vi "EXCEL 画曲线.vi"(8 "错误输入（无错误）":errorcluster, 11 "路径":path) -> (0 "error IO":errorcluster, 2 "XY图":cluster{"X":dbl, "Y":dbl}[](graph))   [LabVIEW 2018]
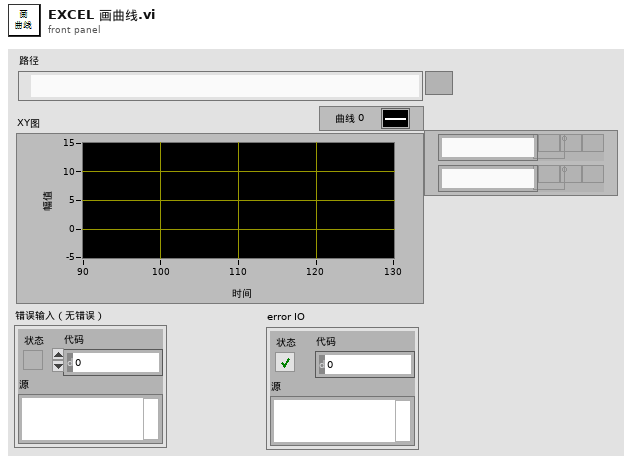
[diagram p1: front panel]
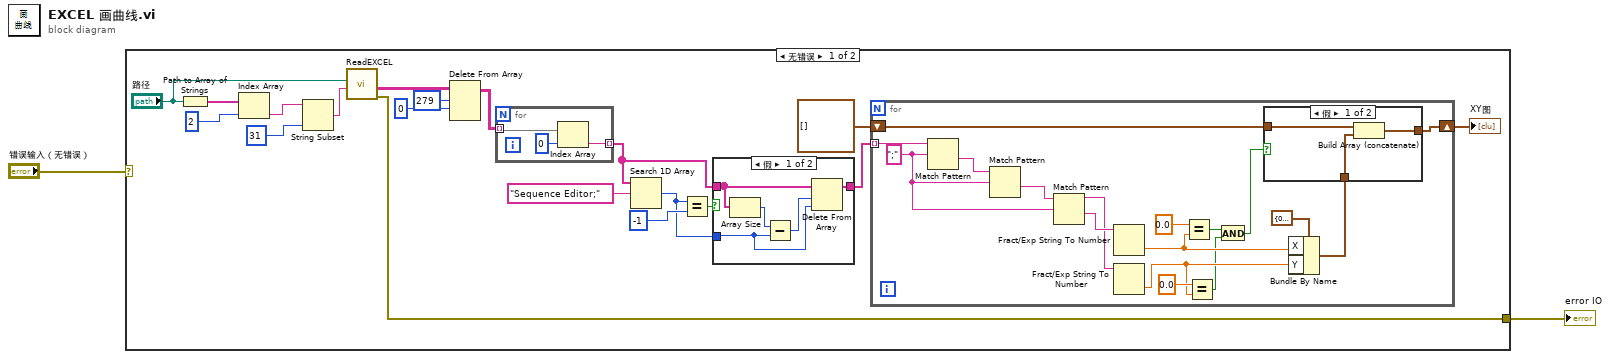
[diagram p0: block diagram]
diagram:
  n1 = case shown="无错误" "错误输入（无错误）" {
    selector: "错误输入（无错误）" -> [_ w52]
    tunnel: [w9 w52] -> w1
    frame No Error {
      n2 = Path to Array of Strings(0:"路径") -> (2:w20:string[])  [unwired: 1 out]
      n3 = Index Array(array=w20, index=2 ("索引")) -> (element=w18:string)
      n4 = String Subset(string=w18, length (rest)=31 ("长度（剩余）")) -> (substring=w16:string)  [unwired: 1 in]
      n5 = call "ReadEXCEL.vi"("EXCEL 标签"=w16, "路径"="路径") -> ("错误输出"=w9:errorcluster, "数据"=w10:string[][])  [unwired: 8 in]
      n6 = Delete From Array(array=w10, length=279 ("长度"), index (row)=0 ("索引 (行)")) -> (array with subset deleted=w13:string[][])  [unwired: 1 in, 1 out]
      n7 = for {
        tunnel: w13 -> [w30] mode=indexing
        tunnel: [w28] -> w6 mode=indexing
        n8 = Index Array(array=w30, index=0 ("索引")) -> (element=w28:string)
      }
      n9 = Search 1D Array(1D array=w6, element="Sequence Editor;" ("元素")) -> (index of element=w3:i32)  [unwired: 1 in]
      n10 = Equal?(x=w3, y=-1) -> (x = y?=w4:bool)
      n11 = case shown="假" w4 {
        tunnel: w6 -> [w25 w27]
        tunnel: [w26 w27] -> w5
        tunnel: w3 -> [w22 _]
        frame False {
          n12 = Array Size(array=w25) -> (size(s)=w24:i32)
          n13 = Subtract(x=w24, y=w22) -> (x-y=w23:i32)
          n14 = Delete From Array(array=w25, length=w23, index=w22) -> (array with subset deleted=w26:string[])  [unwired: 1 out]
        }
        frame True {
        }
      }
      n15 = for {
        tunnel: w5 -> [w47] mode=indexing
        shift-right: [w31] -> w14
        shift-left: cluster{"X":dbl, "Y":dbl}[] [] ("XY图") -> [w43]
        w44 = ";" ("正则表达式")
        n16 = Match Pattern(string=w47, regular expression=w44) -> (after substring=w46:string)  [unwired: 1 in, 3 out]
        n17 = Match Pattern(string=w46, regular expression=w44) -> (after substring=w45:string)  [unwired: 1 in, 3 out]
        n18 = Match Pattern(string=w45, regular expression=w44) -> (before substring=w41:string, after substring=w42:string)  [unwired: 1 in, 2 out]
        n19 = Fract/Exp String To Number(string=w42) -> (number=w39:dbl)  [unwired: 3 in, 1 out]
        n20 = Fract/Exp String To Number(string=w41) -> (number=w36:dbl)  [unwired: 3 in, 1 out]
        n21 = Equal?(x=0.0, y=w39) -> (x = y?=w34:bool)
        n22 = Equal?(x=0.0, y=w36) -> (x = y?=w35:bool)
        n23 = And(x=w34, y=w35) -> (x .and. y?=w32:bool)
        n24 = Bundle By Name(cluster=cluster{"X":dbl, "Y":dbl} {"X"=0.0, "Y"=0.0}, "X"=w39, "Y"=w36) -> (w40:cluster{"X":dbl, "Y":dbl})
        n25 = case shown="假" w32 {
          tunnel: w43 -> [w50 w51]
          tunnel: [w49 w51] -> w31
          tunnel: w40 -> [w48 _]
          frame False {
            n26 = Build Array (concatenate)(w50, w48) -> (w49:cluster{"X":dbl, "Y":dbl}[])
          }
          frame True {
          }
        }
      }
      "XY图" <- w14
    }
    frame Error {
    }
  }
  "error IO" <- w1
